vi "Father MRA Saver.vi"(0 "Frequency Saver?":bool, 1 "Dynamic Data":dynamicdata(waveform), 2 "Feature Index":dynamicdata(waveform), 3 "Session Index":dynamicdata(waveform), 4 "Experiment Index":dynamicdata(waveform)) -> ()   [LabVIEW 2023]
uses:
  <vilib>/express/express shared/transition.llb/Dynamic To Waveform Array.vi
  <vilib>/express/express signal manip/GetorSetDDTAttributes/Set DDT Attributes/SetT0.vi
  <vilib>/express/express shared/transition.llb/Waveform Array To Dynamic.vi
  <vilib>/express/express signal manip/GetorSetDDTAttributes/Set DDT Attributes/Set DDT Properties.xnode
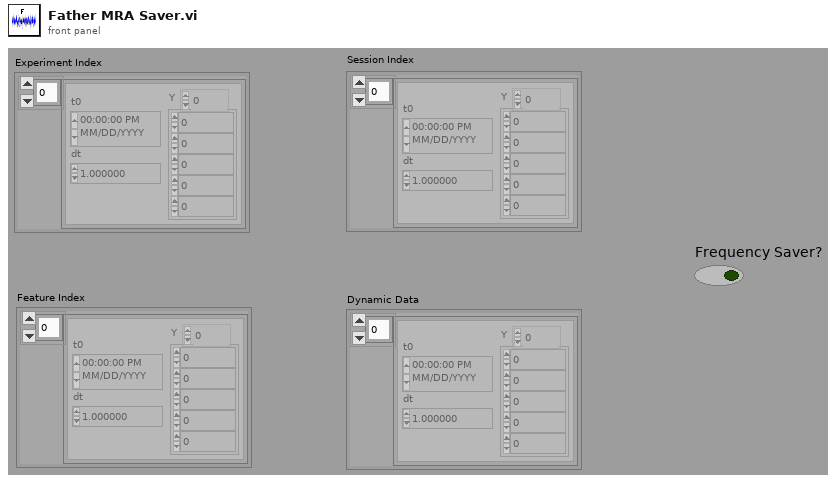
[diagram p1: front panel]
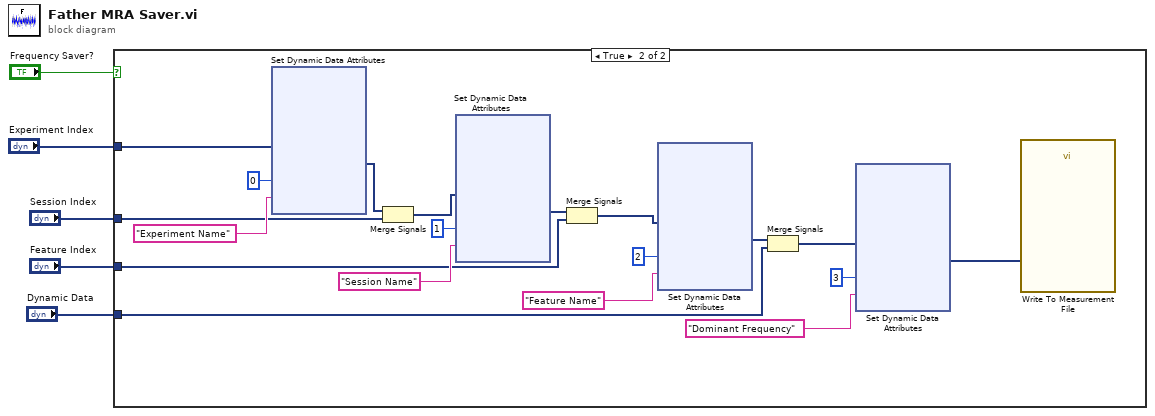
[diagram p0: block diagram]
diagram:
  n1 = case shown="True" "Frequency Saver?" {
    tunnel: "Dynamic Data" -> [_ w7]
    tunnel: "Experiment Index" -> [_ w17]
    tunnel: "Session Index" -> [_ w16]
    tunnel: "Feature Index" -> [_ w8]
    frame False {
    }
    frame True {
      n2 = xnode "Set Dynamic Data Attributes"("Signals In"=w17, "Signal Index"=0, "Signal Name"="Experiment Name") -> ("Signals Out"=w15:dynamicdata)  [unwired: 1 in, 1 out]
      n3 = Merge Signals(w15, w16) -> (w14:dynamicdata)
      n4 = xnode "Set Dynamic Data Attributes"("Signals In"=w14, "Signal Index"=1, "Signal Name"="Session Name") -> ("Signals Out"=w9:dynamicdata)  [unwired: 1 in, 1 out]
      n5 = Merge Signals(w9, w8) -> (w10:dynamicdata)
      n6 = xnode "Set Dynamic Data Attributes"("Signals In"=w10, "Signal Index"=2, "Signal Name"="Feature Name") -> ("Signals Out"=w13:dynamicdata)  [unwired: 1 in, 1 out]
      n7 = Merge Signals(w13, w7) -> (w18:dynamicdata)
      n8 = xnode "Set Dynamic Data Attributes"("Signals In"=w18, "Signal Index"=3, "Signal Name"="Dominant Frequency") -> ("Signals Out"=w6:dynamicdata)  [unwired: 1 in, 1 out]
      n9 = call "Write To Measurement File"("Signals"=w6) -> ()  [unwired: 16 in, 3 out]
    }
  }
